vi "Subpanel UI.vi"(8 "error in (no error)":errorcluster, 10 "Message Queue":refnum<queue>, 11 "Syringe Pump in":refnum<class "Syringe Pump.lvclass">) -> (0 "error out":errorcluster, 3 "Syringe Pump out":refnum<class "Syringe Pump.lvclass">)   [LabVIEW 2020, in "RxnRover.lvlib" / "Syringe Pump.lvclass"]
doc: "The UI that will be inserted into subpanels so data can be displayed to the user. The class will use an internally managed message queue to communicate to it. The user should only communicate to this UI through class methods."
uses:
  Syringe Pump.lvclass
  Sub VIs/Message Queue/Message Cluster.ctl
  Sub VIs/Message Queue/Enqueue Message (Single).vi
  <vilib>/Utility/error.llb/Error Cluster From Error Code.vi
  <vilib>/ErrorRing/Error Ring.xnode
  Sub VIs/Message Queue/test Message Queue.lvlib
panel:
  out "Current Port":u16(knob) scale=1.0..9.0
  out "Syringe":dbl(slide) scale=0.0..50000.0
  out "Inlet":u16
  out "Outlet":u16
  out "Total to Dispense (mL)":dbl
  out "VISA Resource":refnum<visa-resource-name>
  out "Busy?":bool
  out "Error?":bool
  out "Name":string
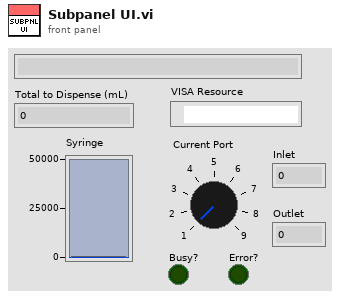
[diagram p1: front panel]
types:
  T1 = typedef "RxnRover.lvlib/Syringe Pump.lvclass/Pump Controller State.ctl" = cluster{"VISA Resource":refnum<visa-resource-name>, "Running":bool, "Running Since":timestamp, "Sampling Rate (sec/sample)":dbl, "Fault":bool, "Total to Dispense (mL)":dbl, "Inlet":u16, "Outlet":u16, "Amount in Syringe (uL)":dbl, "Current Port":u8, "Amount Dispensed (uL)":dbl, "Syringe Volume (uL)":u32}
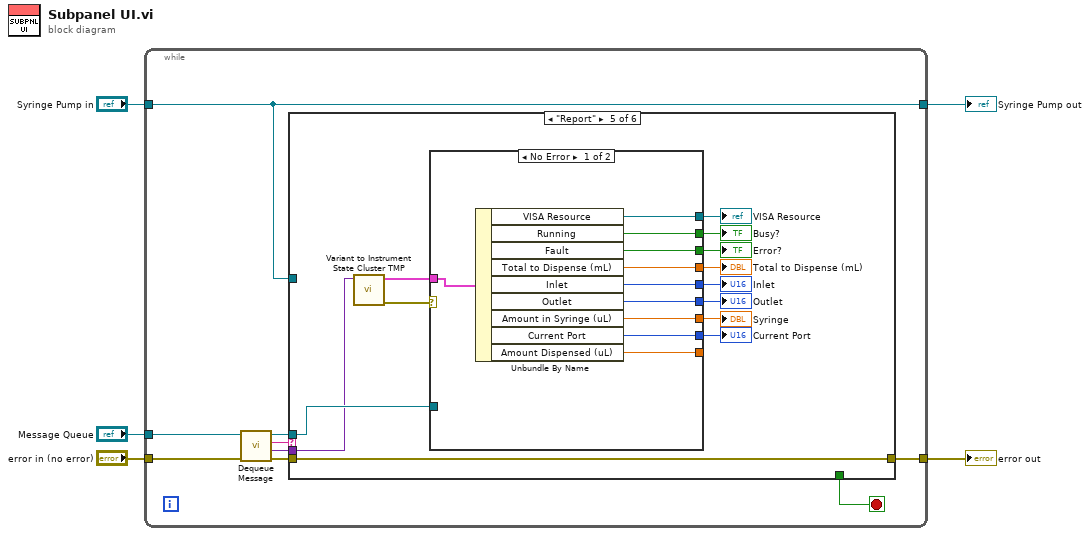
[diagram p0: block diagram]
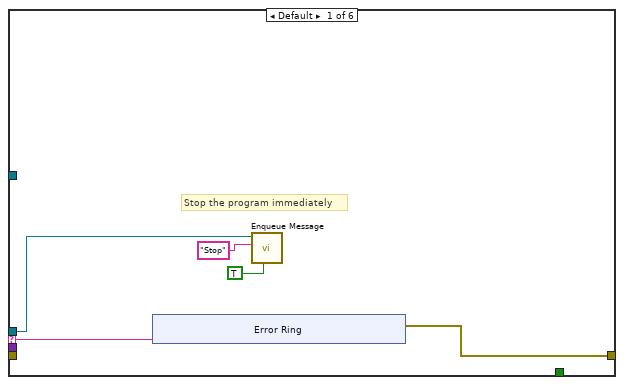
[diagram p2: hidden frame]
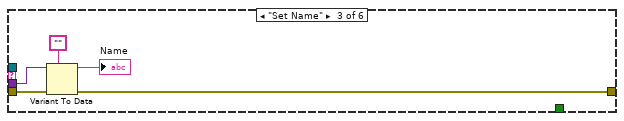
[diagram p4: hidden frame]
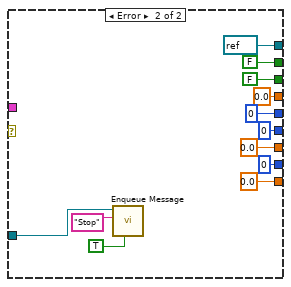
[diagram p6: hidden frame]
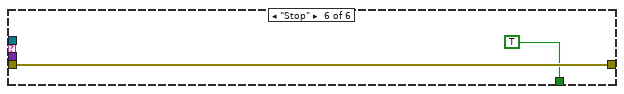
[diagram p7: hidden frame]
diagram:
  n1 = while {
    tunnel: [w6] -> w4
    tunnel: "Syringe Pump in" -> [w6]
    tunnel: [w8] -> w1
    tunnel: "error in (no error)" -> [w14]
    tunnel: "Message Queue" -> [w13]
    stop <- w7 stop-if-true
    n2 = call "Dequeue Message.vi"("error in (no error)"=w14, "Message Queue"=w13) -> ("error out"=w9:errorcluster, "Message Data"=w11:variant, "Message"=w12:string, "dup Message Queue"=w10:refnum<queue>)  [unwired: 6 in]
    n3 = case shown="\"Report\"" w12 {
      selector: w12 -> [w16 _ _ _ _ _]
      tunnel: w11 -> [_ _ w30 _ w43 _]
      tunnel: w10 -> [w17 _ _ _ w44 _]
      tunnel: w9 -> [_ w27 w32 w33 w46 w70]
      tunnel: [w15 w27 w31 w33 w46 w70] -> w8
      tunnel: [_ _ _ _ _ TRUE] -> w7
      tunnel: w6 -> [_ _ _ _ _ _]
      frame Default {
        # "Stop the program immediately"
        n4 = xnode "Error Ring"("parameter 0"=w16) -> ("error out"=w15:errorcluster)
        n5 = call-poly "Enqueue Message.vi"("Priority Message? (F)"=TRUE, "Message"="Stop", "Message Queue"=w17) -> ()  [unwired: 7 in, 2 out]
      }
      frame "--- Copy this frame ---" {
      }
      frame "Set Name" {
        n6 = Variant To Data(error in=w32, type="", Variant=w30) -> (data=→"Name":string, error out=w31:errorcluster)
      }
      frame "Initialize" {
      }
      frame "Report" {
        n7 = call "Variant to Instrument State Cluster TMP.vi"("Message Data"=w43) -> ("error out"=w45:errorcluster, "Instrument State"=w42:T1)  [unwired: 9 in]
        n8 = case shown="No Error" w45 {
          tunnel: w42 -> [w56 _]
          tunnel: w44 -> [_ w68]
          tunnel: [w55 FALSE ("Running")] -> w41
          tunnel: [w54 FALSE ("Fault")] -> w40
          tunnel: [w53 refnum<visa-resource-name> refnum ("VISA Resource")] -> w39
          tunnel: [w52 0.0 ("Total to Dispense (mL)")] -> w38
          tunnel: [w51 u16 0 ("Inlet")] -> w36
          tunnel: [w50 u16 0 ("Outlet")] -> w37
          tunnel: [w49 0.0 ("Amount in Syringe (uL)")] -> w35
          tunnel: [w48 u8 0 ("Current Port")] -> w34
          tunnel: [w47 0.0 ("Amount Dispensed (uL)")] -> _
          frame No Error {
            n9 = Unbundle By Name(w56) -> ("VISA Resource"=w53:refnum<visa-resource-name>, "Running"=w55:bool, "Fault"=w54:bool, "Total to Dispense (mL)"=w52:dbl, "Inlet"=w51:u16, "Outlet"=w50:u16, "Amount in Syringe (uL)"=w49:dbl, "Current Port"=w48:u8, "Amount Dispensed (uL)"=w47:dbl)
          }
          frame Error {
            n10 = call-poly "Enqueue Message.vi"("Priority Message? (F)"=TRUE, "Message"="Stop", "Message Queue"=w68) -> ()  [unwired: 7 in, 2 out]
          }
        }
        "Error?" <- w40
        "Busy?" <- w41
        "VISA Resource" <- w39
        "Total to Dispense (mL)" <- w38
        "Outlet" <- w37
        "Inlet" <- w36
        "Syringe" <- w35
        "Current Port" <- w34
      }
      frame "Stop" {
      }
    }
  }
  "error out" <- w1
  "Syringe Pump out" <- w4
